vi "toFahrenheit.vi"(3 "Celsius temperature":dbl) -> (0 "Fahrenheit temperature":dbl)   [LabVIEW 2014]
doc: "Converts a Celsius temperature reading to a Fahrenheit temperature reading."
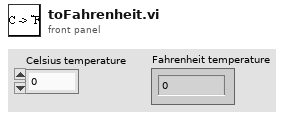
[diagram p1: front panel]
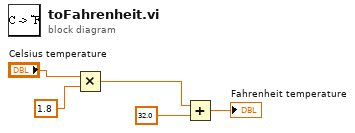
[diagram p0: block diagram]
diagram:
  n1 = Multiply(x="Celsius temperature", y=1.8) -> (x*y=w3:dbl)
  n2 = Add(x=w3, y=32.0) -> (x+y=→"Fahrenheit temperature":dbl)
